vi "dswap.vi"(4 "incy":i32, 6 "incx":i32, 7 "n":i32, 10 "dy":dbl[](array[numeric]), 11 "dx":dbl[](array[numeric])) -> (2 "dy_swaped":dbl[](array[numeric]), 3 "dx_swaped":dbl[](array[numeric]))   [LabVIEW 2014]
panel:
  out "dtemp":dbl
  out "mp1":i32
  out "m":i32=1
  out "iy":i32=1
  out "ix":i32=1
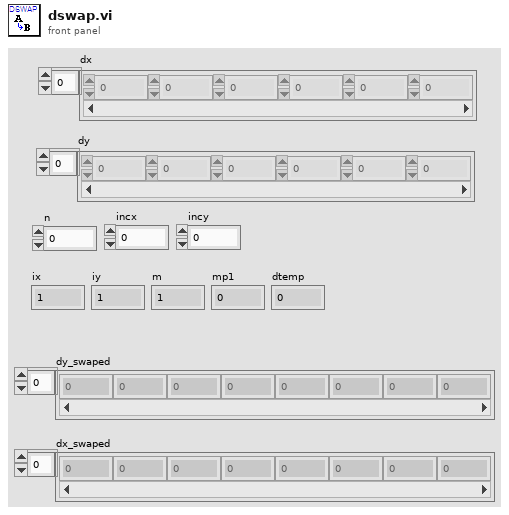
[diagram p1: front panel]
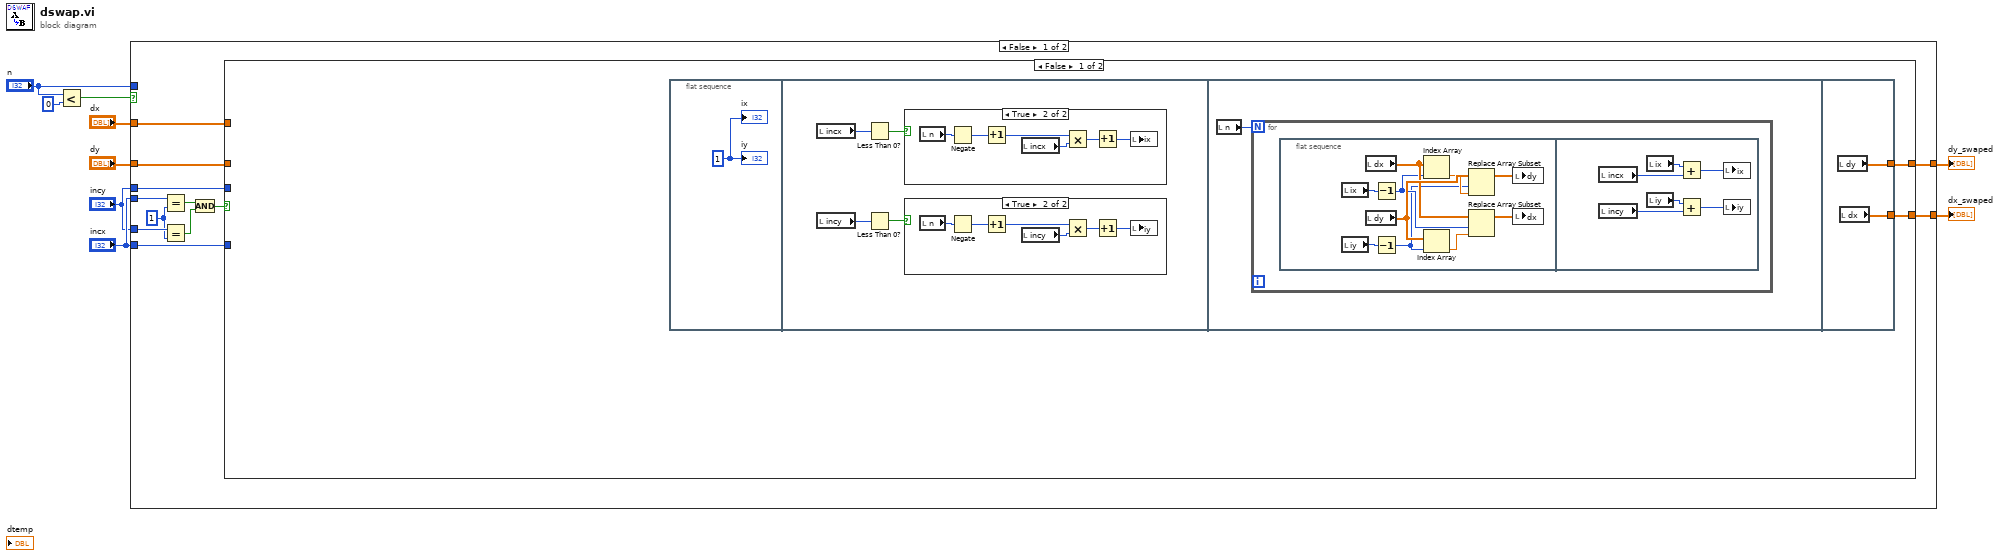
[diagram p0: block diagram]
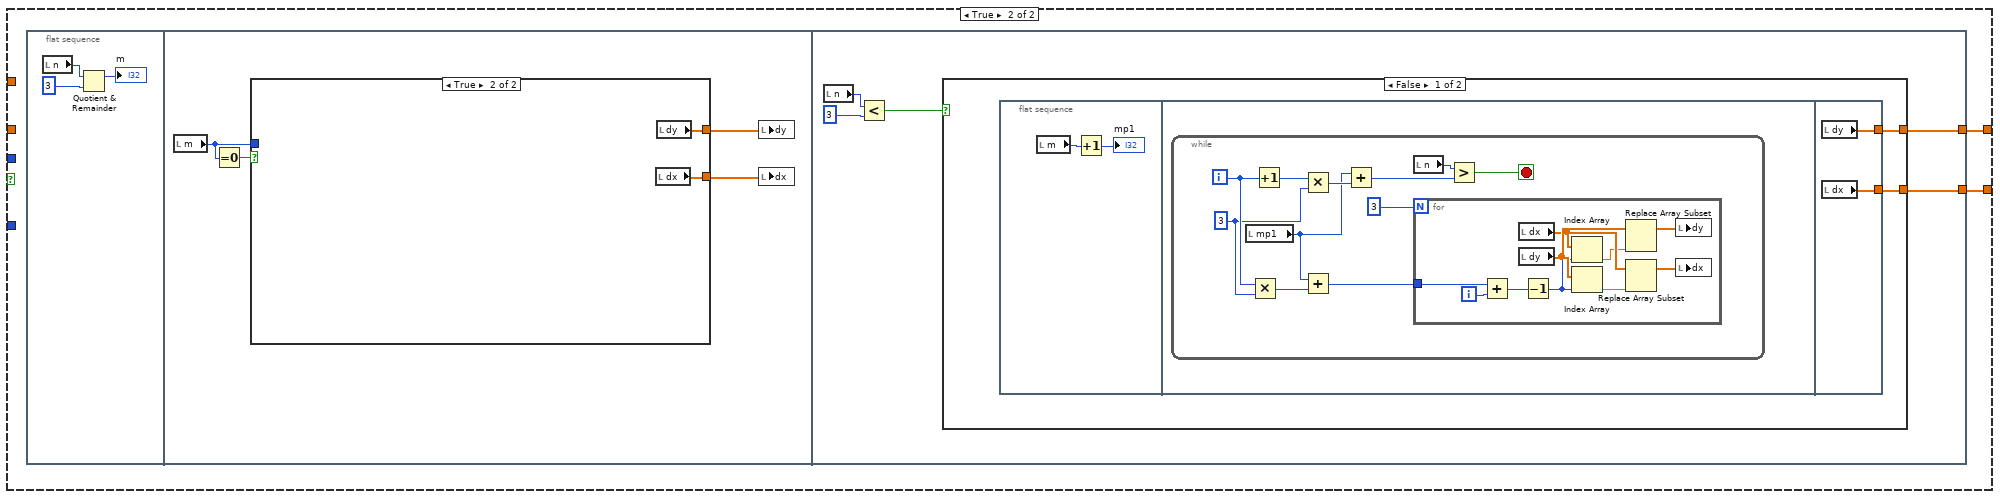
[diagram p4: hidden frame]
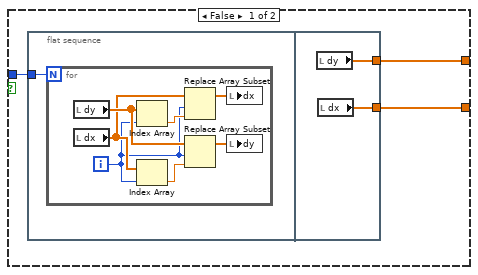
[diagram p5: hidden frame]
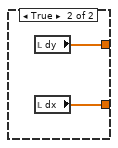
[diagram p6: hidden frame]
diagram:
  n1 = Less?(x="n", y=0) -> (x < y?=w9:bool)
  n2 = case shown="False" w9 {
    tunnel: "dy" -> [w16 w119]
    tunnel: [w11 w119] -> w2
    tunnel: "incx" -> [w21 _]
    tunnel: "dx" -> [w17 w118]
    tunnel: "incy" -> [w20 _]
    tunnel: "n" -> [_ _]
    tunnel: "incx" -> [w19 _]
    tunnel: "incy" -> [w18 _]
    tunnel: [w10 w118] -> w1
    frame False {
      w15 = 1
      n3 = Equal?(x=w21, y=w15) -> (x = y?=w14:bool)
      n4 = Equal?(x=w20, y=w15) -> (x = y?=w13:bool)
      n5 = And(x=w14, y=w13) -> (x .and. y?=w12:bool)
      n6 = case shown="False" w12 {
        tunnel: w19 -> [_ _]
        tunnel: w18 -> [_ _]
        tunnel: w17 -> [_ _]
        tunnel: w16 -> [_ _]
        tunnel: [w23 w61] -> w11
        tunnel: [w22 w60] -> w10
        frame False {
          n7 = flat-sequence {
            tunnel: [w59] -> w23
            tunnel: [w58] -> w22
            frame #0 {
              w24 = 1
              "ix" <- w24
              "iy" <- w24
            }
            frame #1 {
              n8 = local read "incx"() -> (w28:i32)
              n9 = local read "incy"() -> (w25:i32)
              n10 = Less Than 0?(x=w28) -> (x < 0?=w27:bool)
              n11 = Less Than 0?(x=w25) -> (x < 0?=w26:bool)
              n12 = case shown="True" w27 {
                frame False {
                }
                frame True {
                  n13 = local read "n"() -> (w40:i32)
                  n14 = Negate(x=w40) -> (-x=w39:i32)
                  n15 = Increment(x=w39) -> (x+1=w38:i32)
                  n16 = local read "incx"() -> (w37:i32)
                  n17 = Multiply(x=w38, y=w37) -> (x*y=w36:i32)
                  n18 = Increment(x=w36) -> (x+1=w35:i32)
                  n19 = local write "ix"(w35) -> ()
                }
              }
              n20 = case shown="True" w26 {
                frame False {
                }
                frame True {
                  n21 = local read "n"() -> (w34:i32)
                  n22 = Negate(x=w34) -> (-x=w33:i32)
                  n23 = Increment(x=w33) -> (x+1=w32:i32)
                  n24 = local read "incy"() -> (w31:i32)
                  n25 = Multiply(x=w32, y=w31) -> (x*y=w30:i32)
                  n26 = Increment(x=w30) -> (x+1=w29:i32)
                  n27 = local write "iy"(w29) -> ()
                }
              }
            }
            frame #2 {
              n28 = local read "n"() -> (w41:i32)
              n29 = for {
                N: w41 -> [_]
                n30 = flat-sequence {
                  frame #0 {
                    n31 = local read "ix"() -> (w51:i32)
                    n32 = local read "iy"() -> (w50:i32)
                    n33 = local read "dx"() -> (w48:dbl[])
                    n34 = local read "dy"() -> (w49:dbl[])
                    n35 = Decrement(x=w51) -> (x-1=w47:i32)
                    n36 = Decrement(x=w50) -> (x-1=w44:i32)
                    n37 = Index Array(array=w48, index=w47) -> (element=w45:dbl)
                    n38 = Index Array(array=w49, index=w44) -> (element=w46:dbl)
                    n39 = Replace Array Subset(array=w49, new element=w45, index=w44) -> (w43:dbl[])
                    n40 = Replace Array Subset(array=w48, new element=w46, index=w47) -> (w42:dbl[])
                    n41 = local write "dy"(w43) -> ()
                    n42 = local write "dx"(w42) -> ()
                  }
                  frame #1 {
                    n43 = local read "incx"() -> (w56:i32)
                    n44 = local read "incy"() -> (w53:i32)
                    n45 = local read "ix"() -> (w57:i32)
                    n46 = local read "iy"() -> (w52:i32)
                    n47 = Add(x=w57, y=w56) -> (x+y=w55:i32)
                    n48 = Add(x=w52, y=w53) -> (x+y=w54:i32)
                    n49 = local write "ix"(w55) -> ()
                    n50 = local write "iy"(w54) -> ()
                  }
                }
              }
            }
            frame #3 {
              n51 = local read "dy"() -> (w59:dbl[])
              n52 = local read "dx"() -> (w58:dbl[])
            }
          }
        }
        frame True {
          n53 = flat-sequence {
            tunnel: [w85] -> w61
            tunnel: [w84] -> w60
            frame #0 {
              n54 = local read "n"() -> (w63:i32)
              n55 = Quotient & Remainder(x=w63, y=3) -> (x-y*floor(x/y)=→"m":i32)  [unwired: 1 out]
            }
            frame #1 {
              n56 = local read "m"() -> (w67:i32)
              n57 = Equal To 0?(x=w67) -> (x = 0?=w68:bool)
              n58 = case shown="True" w68 {
                tunnel: [w70 w83] -> w66
                tunnel: w67 -> [w71 _]
                tunnel: [w69 w82] -> w65
                frame False {
                  n59 = flat-sequence {
                    tunnel: w71 -> [w72]
                    tunnel: [w81] -> w70
                    tunnel: [w80] -> w69
                    frame #0 {
                      n60 = for {
                        N: w72 -> [_]
                        i -> [w73]
                        n61 = local read "dy"() -> (w79:dbl[])
                        n62 = local read "dx"() -> (w78:dbl[])
                        n63 = Index Array(array=w79, index=w73) -> (element=w77:dbl)
                        n64 = Index Array(array=w78, index=w73) -> (element=w76:dbl)
                        n65 = Replace Array Subset(array=w78, new element=w77, index=w73) -> (w74:dbl[])
                        n66 = Replace Array Subset(array=w79, new element=w76, index=w73) -> (w75:dbl[])
                        n67 = local write "dx"(w74) -> ()
                        n68 = local write "dy"(w75) -> ()
                      }
                    }
                    frame #1 {
                      n69 = local read "dy"() -> (w81:dbl[])
                      n70 = local read "dx"() -> (w80:dbl[])
                    }
                  }
                }
                frame True {
                  n71 = local read "dx"() -> (w82:dbl[])
                  n72 = local read "dy"() -> (w83:dbl[])
                }
              }
              n73 = local write "dy"(w66) -> ()
              n74 = local write "dx"(w65) -> ()
            }
            frame #2 {
              n75 = local read "n"() -> (w88:i32)
              n76 = Less?(x=w88, y=3) -> (x < y?=w87:bool)
              n77 = case shown="False" w87 {
                tunnel: [w90 w117] -> w85
                tunnel: [w89 w116] -> w84
                frame False {
                  n78 = flat-sequence {
                    tunnel: [w115] -> w90
                    tunnel: [w114] -> w89
                    frame #0 {
                      n79 = local read "m"() -> (w92:i32)
                      n80 = Increment(x=w92) -> (x+1=→"mp1":i32)
                    }
                    frame #1 {
                      n81 = while {
                        i -> [w96]
                        stop <- w99 stop-if-true
                        w95 = 3
                        n82 = local read "mp1"() -> (w94:i32)
                        n83 = Multiply(x=w96, y=w95) -> (x*y=w97:i32)
                        n84 = Increment(x=w96) -> (x+1=w103:i32)
                        n85 = Multiply(x=w103, y=w95) -> (x*y=w102:i32)
                        n86 = Add(x=w94, y=w97) -> (x+y=w93:i32)
                        n87 = Add(x=w94, y=w102) -> (x+y=w101:i32)
                        n88 = local read "n"() -> (w100:i32)
                        n89 = for {
                          N: 3 -> [_]
                          tunnel: w93 -> [w107]
                          i -> [w106]
                          n90 = Add(x=w107, y=w106) -> (x+y=w105:i32)
                          n91 = local read "dx"() -> (w112:dbl[])
                          n92 = local read "dy"() -> (w113:dbl[])
                          n93 = Decrement(x=w105) -> (x-1=w104:i32)
                          n94 = Index Array(array=w112, index=w104) -> (element=w110:dbl)
                          n95 = Index Array(array=w113, index=w104) -> (element=w111:dbl)
                          n96 = Replace Array Subset(array=w113, new element=w110) -> (w109:dbl[])  [unwired: 1 in]
                          n97 = Replace Array Subset(array=w112, new element=w111) -> (w108:dbl[])  [unwired: 1 in]
                          n98 = local write "dy"(w109) -> ()
                          n99 = local write "dx"(w108) -> ()
                        }
                        n100 = Greater?(x=w100, y=w101) -> (0:w99:bool)
                      }
                    }
                    frame #2 {
                      n101 = local read "dy"() -> (w115:dbl[])
                      n102 = local read "dx"() -> (w114:dbl[])
                    }
                  }
                }
                frame True {
                  n103 = local read "dy"() -> (w117:dbl[])
                  n104 = local read "dx"() -> (w116:dbl[])
                }
              }
            }
          }
        }
      }
    }
    frame True {
    }
  }
  "dy_swaped" <- w2
  "dx_swaped" <- w1
